vi "Teleop.vi"(10 "Match Info":T1={"Autonomous Elapsed Seconds"=0.0, "TeleOp Elapsed Seconds"=0.0, "Disabled Elapsed Seconds"=0.0, "Visited Autonomous"=FALSE, "Visited TeleOp"=FALSE, "Visited Disabled"=FALSE, "Autonomous Settings"={"Autonomous Style"=enum."Independent", "VI Refnum"=refnum}}, 11 "Call Context":T2) -> ()   [LabVIEW 2015]
doc: "This VI is called for each TeleOp packet received from the DS where the robot is not disabled. It is often used to read from the joysticks and update I/O or to update setpoints for timed control loops. It should complete and return within 20 milliseconds or it may miss DS packets."
uses:
  <vilib>/Rock Robotics/WPI/DriverStation/WPI_DriverStationDerivedRobotMode.ctl
  <vilib>/Rock Robotics/WPI/DriverStation/WPI_DriverStationMatch Info.ctl
  <vilib>/Rock Robotics/Network Tables/SD Read Boolean.vi
  <vilib>/Rock Robotics/Network Tables/SD Read Number.vi
  <vilib>/Rock Robotics/WPI/Utilities/WPI_GetSetVariantRefNum.vi
  <vilib>/Rock Robotics/Network Tables/NT Write Number.vi
  <vilib>/Rock Robotics/Network Tables/SD Write Number.vi
panel:
  out "final_test":dbl
  out "test":dbl
  out "Sample Slider 0":dbl(slide) scale=0.0..5.0
  out "Sample Boolean 1":bool
  out "Sample Boolean 0":bool
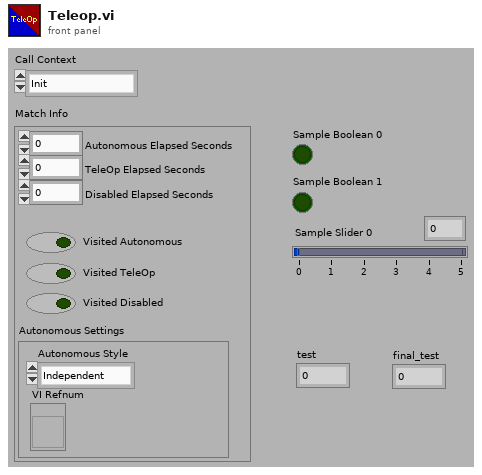
[diagram p1: front panel]
types:
  T1 = typedef "WPI_DriverStationMatch Info.ctl" = cluster{"Autonomous Elapsed Seconds":dbl, "TeleOp Elapsed Seconds":dbl, "Disabled Elapsed Seconds":dbl, "Visited Autonomous":bool, "Visited TeleOp":bool, "Visited Disabled":bool, "Autonomous Settings":cluster{"Autonomous Style":enum16{"Iterative", "Independent"}, "VI Refnum":refnum<vi>}}
  T2 = typedef "WPI_DriverStationDerivedRobotMode.ctl" = enum16{"Init", "Execute", "Stop"}
  T3 = typedef "WPI_EncoderDevRef.ctl" = cluster{"DevStatus":errorcluster, "EncoderIndex":T4, "CounterIndex":T5, "DistancePerCount":dbl, "Decoding Type":T6}
  T4 = typedef "FPGA_EncoderIdx.ctl" = enum8{"Enc 0", "Enc 1", "Enc 2", "Enc 3", "Enc 4", "Enc 5", "Enc 6", "Enc 7", "Invalid"}
  T5 = typedef "FPGA_CounterCtrSystemIndex.ctl" = enum8{"Ctr 0", "Ctr 1", "Ctr 2", "Ctr 3", "Ctr 4", "Ctr 5", "Ctr 6", "Ctr 7", "Invalid"}
  T6 = typedef "WPI_EncoderType.ctl" = enum16{"1x", "2x", "4x"}
  T7 = typedef "WPI_JoystickDevRef.ctl" = cluster{"Device":T8}
  T8 = typedef "WPI_JoystickDeviceEnum.ctl" = enum16{"USB 0", "USB 1", "USB 2", "USB 3", "USB 4", "USB 5"}
  T9 = cluster{"Axes[0]":dbl, "Axes[1]":dbl, "Axes[2]":dbl, "Axes[3]":dbl, "Axes[4]":dbl, "Axes[5]":dbl, "Axes[6]":dbl, "Axes[7]":dbl, "Axes[8]":dbl}
  T10 = typedef "WPI_RobotDriveDevRef.ctl" = cluster{"DevStatus":errorcluster, "Motors[]":T11[], "Square Inputs":bool, "Max Output":dbl}
  T11 = typedef "WPI_MotorControlDeviceRef.ctl" = cluster{"DeviceStatus":errorcluster, "Type":T12, "PWM":cluster{"PWM Channel":T13, "DeadBand":T14}, "CAN":cluster{"Device Number":u8, "Control Mode":T15, "Semaphore":T16, "Max Vout":dbl, "TalonSRX Control Mode":T17}, "Invert":bool}
  T12 = typedef "WPI_MotorControlType.ctl" = enum16{"PWM", "CAN", "CANTalonSRX"}
  T13 = typedef "FPGA_DIOPWMChannel.ctl" = enum8{"PWM 0", "PWM 1", "PWM 2", "PWM 3", "PWM 4", "PWM 5", "PWM 6", "PWM 7", "PWM 8", "PWM 9", "PWM MXP 0", "PWM MXP 1", "PWM MXP 2", "PWM MXP 3", "PWM MXP 4", "PWM MXP 5", "PWM MXP 6", "PWM MXP 7", "PWM MXP 8", "PWM MXP 9", "Invalid"}
  T14 = typedef "WPI_PWMDeadband.ctl" = cluster{"Name":string, "maxPositivePwm":i32, "minPositivePwm":i32, "centerPwm":i32, "maxNegativePwm":i32, "minNegativePwm":i32, "angularRange":u16}
  T15 = typedef "WPI_CANJaguar_ControlMode.ctl" = enum8{"Percent VBus", "Current", "Speed", "Position", "Voltage"}
  T16 = typedef "Semaphore RefNum" = refnum<k1>
  T17 = typedef "WPI_CANTalonSRX_APIControlMode.ctl" = enum8{"Percent VBus", "Speed", "Position", "Slave", "Unchanged / Invalid", "Voltage Compensation", "Current", "Motion Profile"}
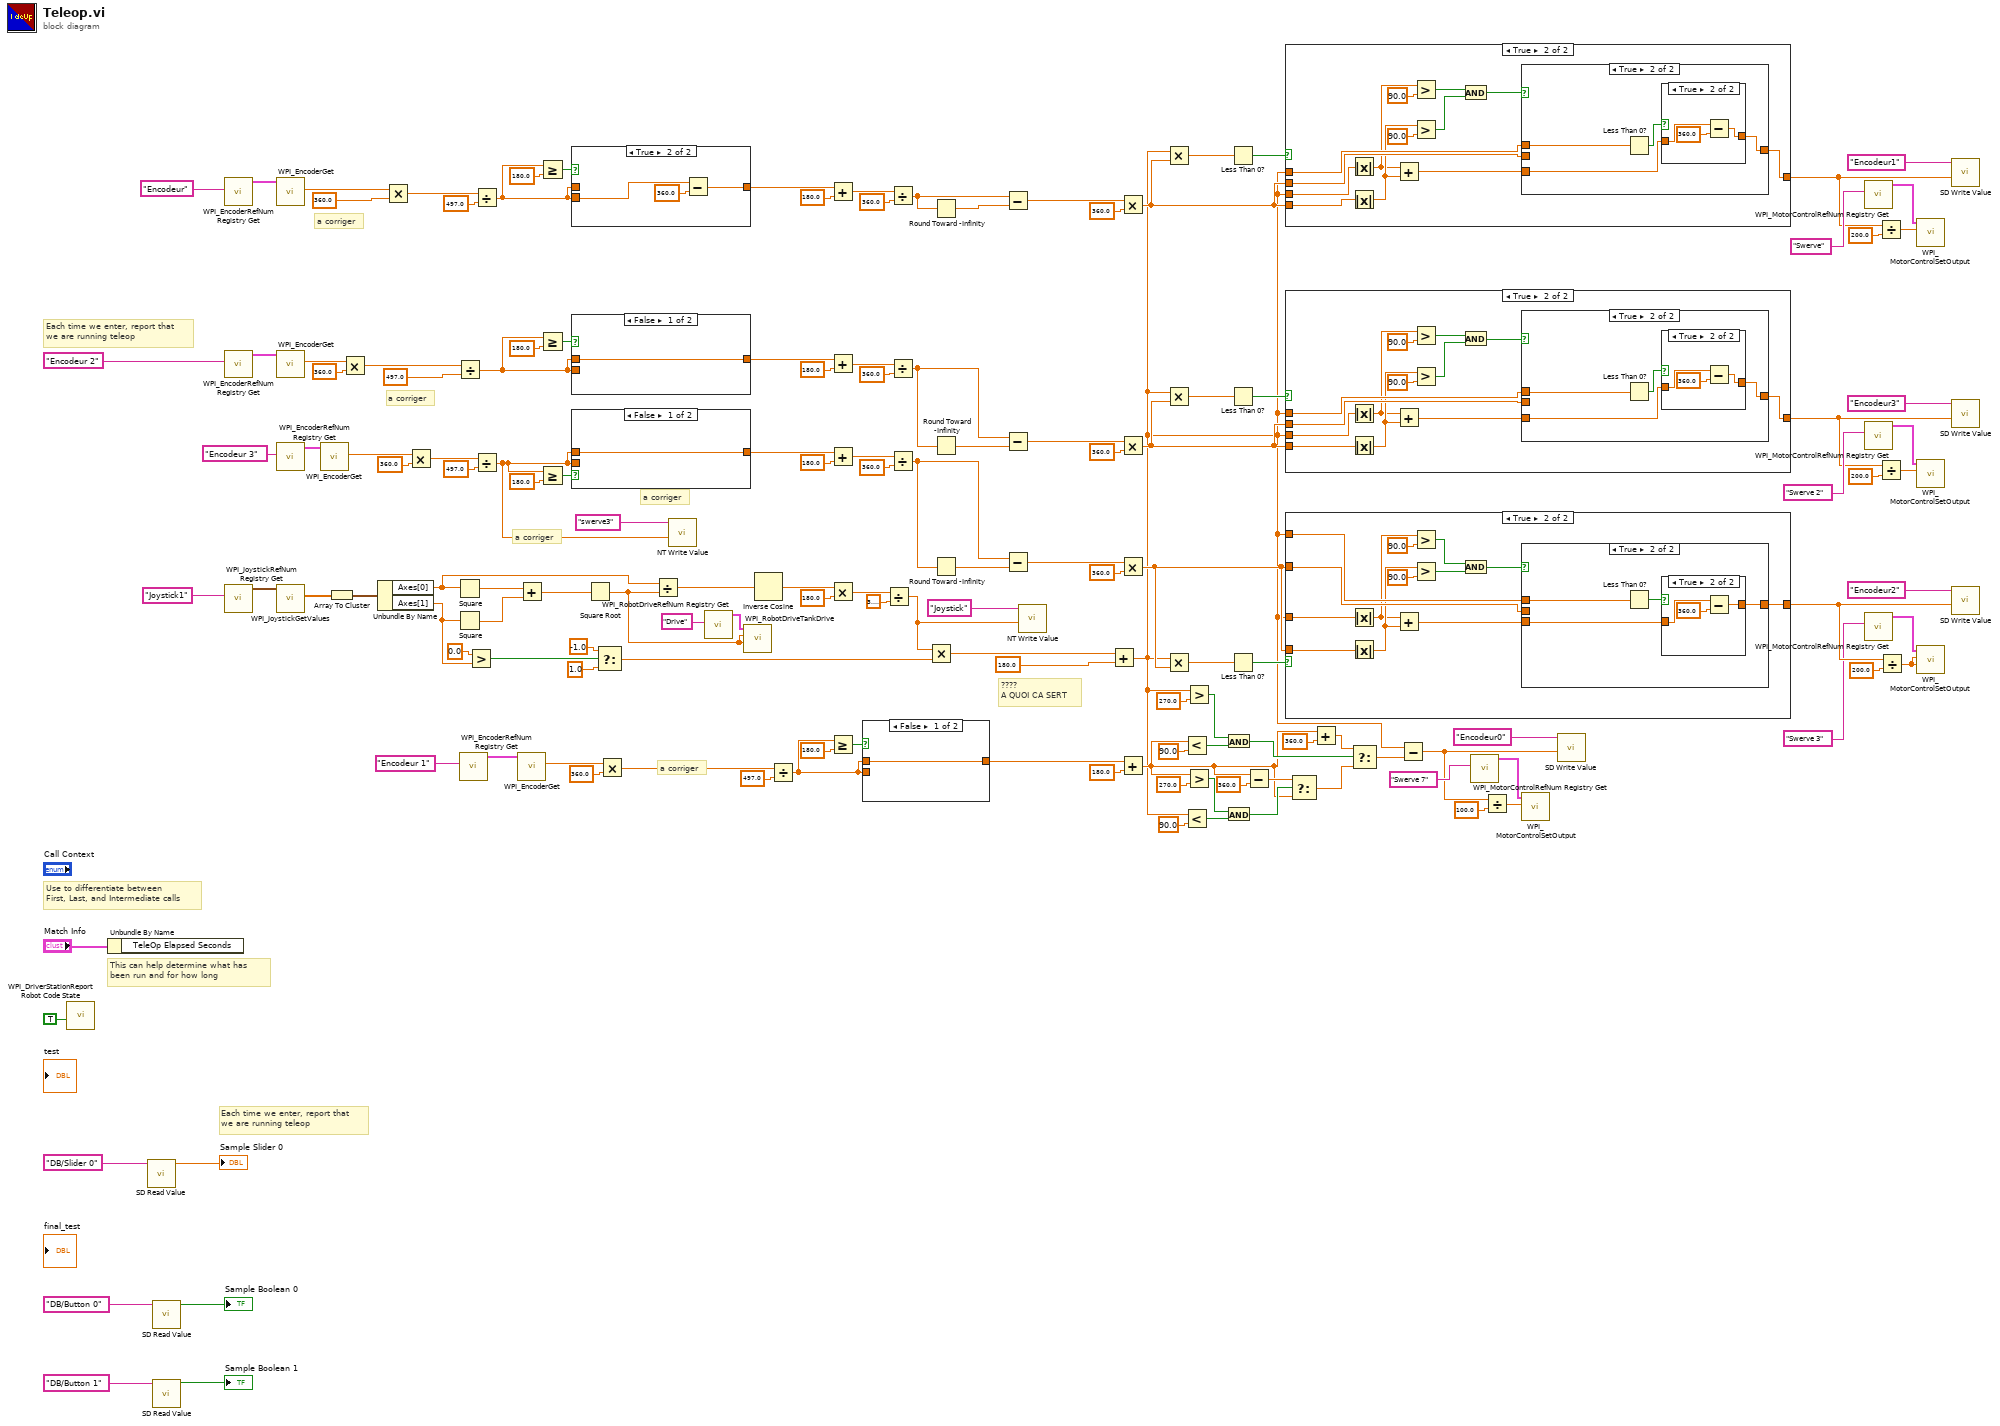
[diagram p0: block diagram]
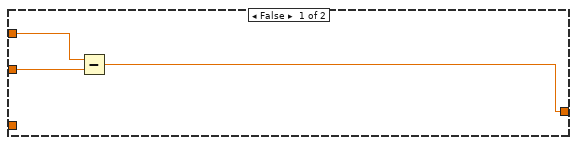
[diagram p2: hidden frame]
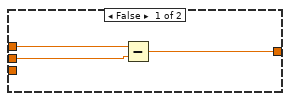
[diagram p3: hidden frame]
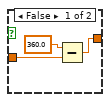
[diagram p4: hidden frame]
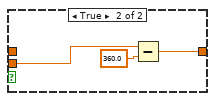
[diagram p5: hidden frame]
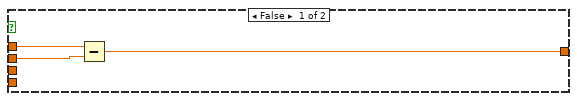
[diagram p6: hidden frame]
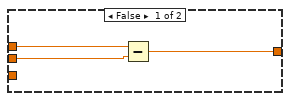
[diagram p7: hidden frame]
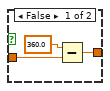
[diagram p8: hidden frame]
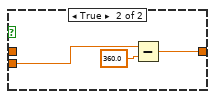
[diagram p9: hidden frame]
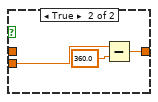
[diagram p10: hidden frame]
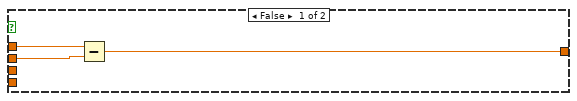
[diagram p11: hidden frame]
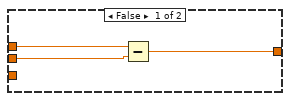
[diagram p12: hidden frame]
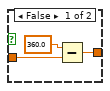
[diagram p13: hidden frame]
diagram:
  # "????\nA QUOI CA SERT"
  # "a corriger"
  # "a corriger"
  # "Each time we enter, report that\nwe are running teleop"
  # "a corriger"
  # "a corriger"
  # "a corriger"
  # "Each time we enter, report that\nwe are running teleop"
  # "Use to differentiate between\nFirst, Last, and Intermediate calls"
  # "This can help determine what has\nbeen run and for how long"
  n1 = call <vilib>:"WPI_DriverStationReport Robot Code State.vi"("TeleOp"=TRUE ("Autonomous")) -> ()  [unwired: 10 in, 1 out]
  n2 = Unbundle By Name("Match Info") -> ()  [unwired: 1 out]
  n3 = call-poly <vilib>:"SD Read Value.vi"("Name"="DB/Slider 0" ("refnum name")) -> ("Numeric"=→"Sample Slider 0":dbl)  [unwired: 8 in, 2 out]
  n4 = call-poly <vilib>:"SD Read Value.vi"("Name"="DB/Button 0" ("refnum name")) -> ("Boolean"=→"Sample Boolean 0":bool)  [unwired: 8 in, 2 out]
  n5 = call-poly <vilib>:"SD Read Value.vi"("Name"="DB/Button 1" ("refnum name")) -> ("Boolean"=→"Sample Boolean 1":bool)  [unwired: 8 in, 2 out]
  n6 = call <vilib>:"WPI_EncoderRefNum Registry Get.vi"("refnum name"="Encodeur") -> ("EncoderDevRef"=w133:T3)  [unwired: 9 in, 1 out]
  n7 = call <vilib>:"WPI_EncoderRefNum Registry Get.vi"("refnum name"="Encodeur 2") -> ("EncoderDevRef"=w81:T3)  [unwired: 9 in, 1 out]
  n8 = call <vilib>:"WPI_JoystickRefNum Registry Get.vi"("refnum name"="Joystick1") -> ("JoystickDevRef"=w140:T7)  [unwired: 9 in, 1 out]
  n9 = call <vilib>:"WPI_EncoderGet.vi"("EncoderDevRef"=w133) -> ("Distance"=w98:dbl)  [unwired: 5 in, 5 out]
  n10 = call <vilib>:"WPI_EncoderGet.vi"("EncoderDevRef"=w81) -> ("Distance"=w60:dbl)  [unwired: 5 in, 5 out]
  n11 = call <vilib>:"WPI_EncoderRefNum Registry Get.vi"("refnum name"="Encodeur 3") -> ("EncoderDevRef"=w58:T3)  [unwired: 9 in, 1 out]
  n12 = call <vilib>:"WPI_JoystickGetValues.vi"("JoystickDevRef"=w140) -> ("Axes"=w138:dbl[])  [unwired: 6 in, 4 out]
  n13 = call <vilib>:"WPI_EncoderGet.vi"("EncoderDevRef"=w58) -> ("Distance"=w39:dbl)  [unwired: 5 in, 5 out]
  n14 = Array To Cluster(array=w138) -> (cluster=w137:T9)
  n15 = Multiply(x=w60, y=360.0) -> (x*y=w79:dbl)
  n16 = Unbundle By Name(w137) -> ("Axes[0]"=w99:dbl, "Axes[1]"=w4:dbl)
  n17 = Multiply(x=w98, y=360.0) -> (x*y=w124:dbl)
  n18 = Multiply(x=w39, y=360.0) -> (x*y=w56:dbl)
  n19 = Square(x=w99) -> (x^2=w131:dbl)
  n20 = Square(x=w4) -> (x^2=w132:dbl)
  n21 = Divide(x=w79, y=497.0) -> (x/y=w73:dbl)
  n22 = call <vilib>:"WPI_EncoderRefNum Registry Get.vi"("refnum name"="Encodeur 1") -> ("EncoderDevRef"=w96:T3)  [unwired: 9 in, 1 out]
  n23 = Greater?(x=0.0, y=w4) -> (0:w7:bool)
  n24 = Divide(x=w124, y=497.0) -> (x/y=w117:dbl)
  n25 = Divide(x=w56, y=497.0) -> (x/y=w10:dbl)
  n26 = Add(x=w131, y=w132) -> (x+y=w130:dbl)
  n27 = call <vilib>:"WPI_EncoderGet.vi"("EncoderDevRef"=w96) -> ("Distance"=w87:dbl)  [unwired: 5 in, 5 out]
  n28 = Greater Or Equal?(x=w117, y=180.0) -> (x >= y?=w118:bool)
  n29 = Greater Or Equal?(x=w73, y=180.0) -> (x >= y?=w74:bool)
  n30 = Greater Or Equal?(x=w10, y=180.0) -> (x >= y?=w52:bool)
  n31 = case shown="True" w118 {
    tunnel: w117 -> [_ w151]
    tunnel: [w149 w150] -> w115
    tunnel: w117 -> [w149 _]
    frame False {
    }
    frame True {
      n32 = Subtract(x=w151, y=360.0) -> (x-y=w150:dbl)
    }
  }
  n33 = case shown="False" w74 {
    tunnel: w73 -> [_ w155]
    tunnel: [w153 w154] -> w72
    tunnel: w73 -> [w153 _]
    frame False {
    }
    frame True {
      n34 = Subtract(x=w155, y=360.0) -> (x-y=w154:dbl)
    }
  }
  n35 = case shown="False" w52 {
    tunnel: w10 -> [_ w159]
    tunnel: [w157 w158] -> w51
    tunnel: w10 -> [w157 _]
    frame False {
    }
    frame True {
      n36 = Subtract(x=w159, y=360.0) -> (x-y=w158:dbl)
    }
  }
  n37 = Square Root(x=w130) -> (sqrt(x)=w105:dbl)
  n38 = Select(t=-1.0, s=w7, f=1.0) -> (s? t:f=w3:dbl)
  n39 = Multiply(x=w87, y=360.0) -> (x*y=w94:dbl)
  n40 = Divide(x=w99, y=w105) -> (x/y=w129:dbl)
  n41 = call-poly <vilib>:"NT Write Value.vi"("Numeric"=w10, "Name"="swerve3") -> ()  [unwired: 9 in, 1 out]
  n42 = call <vilib>:"WPI_RobotDriveRefNum Registry Get.vi"("refnum name"="Drive") -> ("RobotDriveDevRef"=w106:T10)  [unwired: 9 in, 1 out]
  n43 = call <vilib>:"WPI_RobotDriveTankDrive.vi"("Right axis value"=w105, "Left axis value"=w105, "RobotDriveDevRef"=w106) -> ()  [unwired: 6 in, 3 out]
  n44 = Inverse Cosine(1:w129) -> (0:w120:dbl)
  n45 = Divide(x=w94, y=497.0) -> (x/y=w90:dbl)
  n46 = Add(x=w115, y=180.0) -> (x+y=w113:dbl)
  n47 = Add(x=w72, y=180.0) -> (x+y=w70:dbl)
  n48 = Add(x=w51, y=180.0) -> (x+y=w49:dbl)
  n49 = Multiply(x=w120, y=180.0) -> (x*y=w127:dbl)
  n50 = Greater Or Equal?(x=w90, y=180.0) -> (x >= y?=w91:bool)
  n51 = case shown="False" w91 {
    tunnel: w90 -> [_ w163]
    tunnel: [w161 w162] -> w89
    tunnel: w90 -> [w161 _]
    frame False {
    }
    frame True {
      n52 = Subtract(x=w163, y=360.0) -> (x-y=w162:dbl)
    }
  }
  n53 = Divide(x=w127, y=3.141592653589793) -> (x/y=w2:dbl)
  n54 = Divide(x=w113, y=360.0) -> (x/y=w110:dbl)
  n55 = Divide(x=w70, y=360.0) -> (x/y=w67:dbl)
  n56 = Divide(x=w49, y=360.0) -> (x/y=w46:dbl)
  n57 = Multiply(x=w2, y=w3) -> (x*y=w1:dbl)
  n58 = Round Toward -Infinity(1:w110) -> (0:w111:dbl)
  n59 = Round Toward -Infinity(1:w67) -> (0:w68:dbl)
  n60 = Round Toward -Infinity(1:w46) -> (0:w47:dbl)
  n61 = Subtract(x=w110, y=w111) -> (x-y=w108:dbl)
  n62 = Subtract(x=w67, y=w68) -> (x-y=w65:dbl)
  n63 = Subtract(x=w46, y=w47) -> (x-y=w44:dbl)
  n64 = call-poly <vilib>:"NT Write Value.vi"("Numeric"=w2, "Name"="Joystick") -> ()  [unwired: 9 in, 1 out]
  n65 = Add(x=w1, y=180.0) -> (x+y=w17:dbl)
  n66 = Multiply(x=w108, y=360.0) -> (x*y=w102:dbl)
  n67 = Multiply(x=w65, y=360.0) -> (x*y=w62:dbl)
  n68 = Multiply(x=w44, y=360.0) -> (x*y=w41:dbl)
  n69 = Add(x=w89, y=180.0) -> (x+y=w22:dbl)
  n70 = Multiply(x=w17, y=w102) -> (x*y=w104:dbl)
  n71 = Multiply(x=w17, y=w62) -> (x*y=w64:dbl)
  n72 = Multiply(x=w17, y=w41) -> (x*y=w43:dbl)
  n73 = Less?(x=w22, y=90.0) -> (x < y?=w25:bool)
  n74 = Less?(x=w17, y=90.0) -> (x < y?=w33:bool)
  n75 = Greater?(x=w17, y=270.0) -> (0:w27:bool)
  n76 = Greater?(x=w22, y=270.0) -> (0:w35:bool)
  n77 = And(x=w27, y=w25) -> (x .and. y?=w24:bool)
  n78 = And(x=w35, y=w33) -> (x .and. y?=w31:bool)
  n79 = Less Than 0?(x=w104) -> (x < 0?=w103:bool)
  n80 = Less Than 0?(x=w64) -> (x < 0?=w63:bool)
  n81 = Less Than 0?(x=w43) -> (x < 0?=w42:bool)
  n82 = Subtract(x=w22, y=360.0) -> (x-y=w29:dbl)
  n83 = case shown="True" w103 {
    tunnel: [w167 w180] -> w101
    tunnel: w17 -> [w166 w179]
    tunnel: w102 -> [w165 w178]
    tunnel: w17 -> [_ w172]
    tunnel: w102 -> [_ w171]
    frame False {
      n84 = Subtract(x=w166, y=w165) -> (x-y=w167:dbl)
    }
    frame True {
      n85 = Absolute Value(x=w172) -> (abs(x)=w169:dbl)
      n86 = Absolute Value(x=w171) -> (abs(x)=w170:dbl)
      n87 = Add(x=w169, y=w170) -> (x+y=w168:dbl)
      n88 = Greater?(x=w169, y=90.0) -> (0:w174:bool)
      n89 = Greater?(x=w170, y=90.0) -> (0:w173:bool)
      n90 = And(x=w174, y=w173) -> (x .and. y?=w177:bool)
      n91 = case shown="True" w177 {
        tunnel: [w181 w186] -> w180
        tunnel: w179 -> [w183 w185]
        tunnel: w178 -> [w182 _]
        tunnel: w168 -> [_ w184]
        frame False {
          n92 = Subtract(x=w183, y=w182) -> (x-y=w181:dbl)
        }
        frame True {
          n93 = Less Than 0?(x=w185) -> (x < 0?=w187:bool)
          n94 = case shown="True" w187 {
            tunnel: [w190 w193] -> w186
            tunnel: w184 -> [w188 w191]
            frame False {
              n95 = Subtract(x=360.0 ("y"), y=w188) -> (x-y=w190:dbl)
            }
            frame True {
              n96 = Subtract(x=w191, y=360.0 ("x")) -> (x-y=w193:dbl)
            }
          }
        }
      }
    }
  }
  n97 = case shown="True" w63 {
    tunnel: [w196 w209] -> w61
    tunnel: w17 -> [w195 w208]
    tunnel: w62 -> [w194 w207]
    tunnel: w17 -> [_ w201]
    tunnel: w62 -> [_ w200]
    frame False {
      n98 = Subtract(x=w195, y=w194) -> (x-y=w196:dbl)
    }
    frame True {
      n99 = Absolute Value(x=w201) -> (abs(x)=w198:dbl)
      n100 = Absolute Value(x=w200) -> (abs(x)=w199:dbl)
      n101 = Add(x=w198, y=w199) -> (x+y=w197:dbl)
      n102 = Greater?(x=w198, y=90.0) -> (0:w203:bool)
      n103 = Greater?(x=w199, y=90.0) -> (0:w202:bool)
      n104 = And(x=w203, y=w202) -> (x .and. y?=w206:bool)
      n105 = case shown="True" w206 {
        tunnel: [w210 w215] -> w209
        tunnel: w208 -> [w212 w214]
        tunnel: w207 -> [w211 _]
        tunnel: w197 -> [_ w213]
        frame False {
          n106 = Subtract(x=w212, y=w211) -> (x-y=w210:dbl)
        }
        frame True {
          n107 = Less Than 0?(x=w214) -> (x < 0?=w216:bool)
          n108 = case shown="True" w216 {
            tunnel: [w219 w222] -> w215
            tunnel: w213 -> [w217 w220]
            frame False {
              n109 = Subtract(x=360.0 ("y"), y=w217) -> (x-y=w219:dbl)
            }
            frame True {
              n110 = Subtract(x=w220, y=360.0 ("x")) -> (x-y=w222:dbl)
            }
          }
        }
      }
    }
  }
  n111 = case shown="True" w42 {
    tunnel: [w225 w238] -> w40
    tunnel: w17 -> [w224 w237]
    tunnel: w41 -> [w223 w236]
    tunnel: w17 -> [_ w230]
    tunnel: w41 -> [_ w229]
    frame False {
      n112 = Subtract(x=w224, y=w223) -> (x-y=w225:dbl)
    }
    frame True {
      n113 = Absolute Value(x=w230) -> (abs(x)=w227:dbl)
      n114 = Absolute Value(x=w229) -> (abs(x)=w228:dbl)
      n115 = Add(x=w227, y=w228) -> (x+y=w226:dbl)
      n116 = Greater?(x=w227, y=90.0) -> (0:w232:bool)
      n117 = Greater?(x=w228, y=90.0) -> (0:w231:bool)
      n118 = And(x=w232, y=w231) -> (x .and. y?=w235:bool)
      n119 = case shown="True" w235 {
        tunnel: [w239 w244] -> w238
        tunnel: w237 -> [w241 w243]
        tunnel: w236 -> [w240 _]
        tunnel: w226 -> [_ w242]
        frame False {
          n120 = Subtract(x=w241, y=w240) -> (x-y=w239:dbl)
        }
        frame True {
          n121 = Less Than 0?(x=w243) -> (x < 0?=w245:bool)
          n122 = case shown="True" w245 {
            tunnel: [w248 w251] -> w244
            tunnel: w242 -> [w246 w249]
            frame False {
              n123 = Subtract(x=360.0 ("y"), y=w246) -> (x-y=w248:dbl)
            }
            frame True {
              n124 = Subtract(x=w249, y=360.0 ("x")) -> (x-y=w251:dbl)
            }
          }
        }
      }
    }
  }
  n125 = Select(t=w29, s=w31, f=w22) -> (s? t:f=w20:dbl)
  n126 = Add(x=w22, y=360.0) -> (x+y=w21:dbl)
  n127 = Select(t=w21, s=w24, f=w20) -> (s? t:f=w16:dbl)
  n128 = Subtract(x=w17, y=w16) -> (x-y=w15:dbl)
  n129 = call <vilib>:"WPI_MotorControlRefNum Registry Get.vi"("refnum name"="Swerve 7") -> ("MotorControlDevRef"=w85:T11)  [unwired: 9 in, 1 out]
  n130 = Divide(x=w15, y=100.0) -> (x/y=w18:dbl)
  n131 = call <vilib>:"WPI_MotorControlSetOutput.vi"("Output"=w18, "MotorControlDevRef"=w85) -> ()  [unwired: 7 in, 3 out]
  n132 = call-poly <vilib>:"SD Write Value.vi"("Numeric"=w15, "Name"="Encodeur0") -> ()  [unwired: 8 in, 2 out]
  n133 = call <vilib>:"WPI_MotorControlRefNum Registry Get.vi"("refnum name"="Swerve") -> ("MotorControlDevRef"=w135:T11)  [unwired: 9 in, 1 out]
  n134 = call <vilib>:"WPI_MotorControlRefNum Registry Get.vi"("refnum name"="Swerve 2") -> ("MotorControlDevRef"=w83:T11)  [unwired: 9 in, 1 out]
  n135 = call <vilib>:"WPI_MotorControlRefNum Registry Get.vi"("refnum name"="Swerve 3") -> ("MotorControlDevRef"=w37:T11)  [unwired: 9 in, 1 out]
  n136 = Divide(x=w101, y=200.0) -> (x/y=w121:dbl)
  n137 = Divide(x=w61, y=200.0) -> (x/y=w76:dbl)
  n138 = Divide(x=w40, y=200.0) -> (x/y=w38:dbl)
  n139 = call <vilib>:"WPI_MotorControlSetOutput.vi"("Output"=w121, "MotorControlDevRef"=w135) -> ()  [unwired: 7 in, 3 out]
  n140 = call <vilib>:"WPI_MotorControlSetOutput.vi"("Output"=w76, "MotorControlDevRef"=w83) -> ()  [unwired: 7 in, 3 out]
  n141 = call <vilib>:"WPI_MotorControlSetOutput.vi"("Sync Group / Parameter Slot"=w38, "Output"=w38, "MotorControlDevRef"=w37) -> ()  [unwired: 6 in, 3 out]
  n142 = call-poly <vilib>:"SD Write Value.vi"("Numeric"=w101, "Name"="Encodeur1") -> ()  [unwired: 8 in, 2 out]
  n143 = call-poly <vilib>:"SD Write Value.vi"("Numeric"=w61, "Name"="Encodeur3") -> ()  [unwired: 8 in, 2 out]
  n144 = call-poly <vilib>:"SD Write Value.vi"("Numeric"=w40, "Name"="Encodeur2") -> ()  [unwired: 8 in, 2 out]
